vi "Begin.vi"(8 "error in":errorcluster) -> (0 "error out":errorcluster)   [LabVIEW 2017]
doc: "Called before other user functions, this VI is expected to open initial I/O refnums, load in file data, and do all program initialization. Notice that the <B>error out</B> terminal is simply used for data flow. Wiring it to other structures or subVIs ensures that this VI runs first."
uses:
  <vilib>/Rock Robotics/WPI/DriverStation/WPI_DriverStationRobotMode2.ctl
  <vilib>/Rock Robotics/SystemInterfaces/DIO/FPGA_DIOPWMChannel.ctl
  <vilib>/Rock Robotics/WPI/Joystick/WPI_JoystickDeviceEnum.ctl
  Robot Global Data.vi
  <vilib>/Rock Robotics/Network Tables/NT Write String Array.vi
  <vilib>/Rock Robotics/WPI/RobotDrive/WPI_RobotDriveOpen2MotorWithSPARK.vi
  <vilib>/Rock Robotics/WPI/RobotDrive/WPI_RobotDriveOpen4MotorWithSPARK.vi
  <vilib>/Rock Robotics/WPI/MotorControl/WPI_MotorControlOpen SPARK.vi
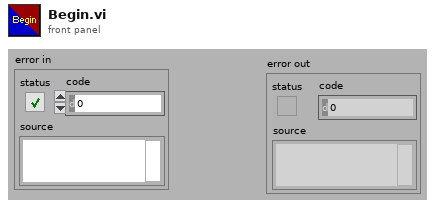
[diagram p1: front panel]
types:
  T1 = typedef "FPGA_DIOPWMChannel.ctl" = enum8{"PWM 0", "PWM 1", "PWM 2", "PWM 3", "PWM 4", "PWM 5", "PWM 6", "PWM 7", "PWM 8", "PWM 9", "PWM MXP 0", "PWM MXP 1", "PWM MXP 2", "PWM MXP 3", "PWM MXP 4", "PWM MXP 5", "PWM MXP 6", "PWM MXP 7", "PWM MXP 8", "PWM MXP 9", "Invalid"}
  T2 = typedef "WPI_JoystickDeviceEnum.ctl" = enum16{"USB 0", "USB 1", "USB 2", "USB 3", "USB 4", "USB 5"}
  T3 = typedef "WPI_DriverStationRobotMode2.ctl" = enum16{"Autonomous Disabled", "Autonomous Enabled", "Teleop Disabled", "Teleop Enabled", "Disconnected", "Finish", "Test Disabled", "Test Enabled", "Emergency Stopped"}
  T4 = typedef "WPI_MotorControlDeviceRef.ctl" = cluster{"DeviceStatus":errorcluster, "Type":T5, "PWM":cluster{"PWM Channel":T1, "DeadBand":T6}, "CAN":cluster{"Device Number":u8, "SetOutput VI Ref":variant, "GetOutput VI Ref":variant, "Enable VI Ref":variant, "Disable VI Ref":variant, "Data":variant}, "Invert":bool, "DIO PWM":cluster{"PWM \"Enable\" Channel":T1, "DIOChannel":T7, "PWM Rate":dbl}}
  T5 = typedef "WPI_MotorControlType.ctl" = enum16{"PWM", "CAN", "DIO PWM"}
  T6 = typedef "WPI_PWMDeadband.ctl" = cluster{"Name":string, "maxPositivePwm":i32, "minPositivePwm":i32, "centerPwm":i32, "maxNegativePwm":i32, "minNegativePwm":i32, "angularRange":u16}
  T7 = typedef "FPGA_DIOChannel.ctl" = enum8{"DIO 0", "DIO 1", "DIO 2", "DIO 3", "DIO 4", "DIO 5", "DIO 6", "DIO 7", "DIO 8", "DIO 9", "DIO MXP 0", "DIO MXP 1", "DIO MXP 2", "DIO MXP 3", "DIO MXP 4", "DIO MXP 5", "DIO MXP 6", "DIO MXP 7", "DIO MXP 8", "DIO MXP 9", "DIO MXP 10", "DIO MXP 11", "DIO MXP 12", "DIO MXP 13", "DIO MXP 14", "DIO MXP 15", "SPI Port CS1", "SPI Port CS2", "SPI Port CS3", "SPI Port MISO", "SPI Port MOSI", "Invalid"}
  T8 = typedef "WPI_RobotDriveDevRef.ctl" = cluster{"DevStatus":errorcluster, "Motors[]":T4[], "Square Inputs":bool, "Max Output":dbl}
  T9 = typedef "WPI_JoystickDevRef.ctl" = cluster{"Device":T2}
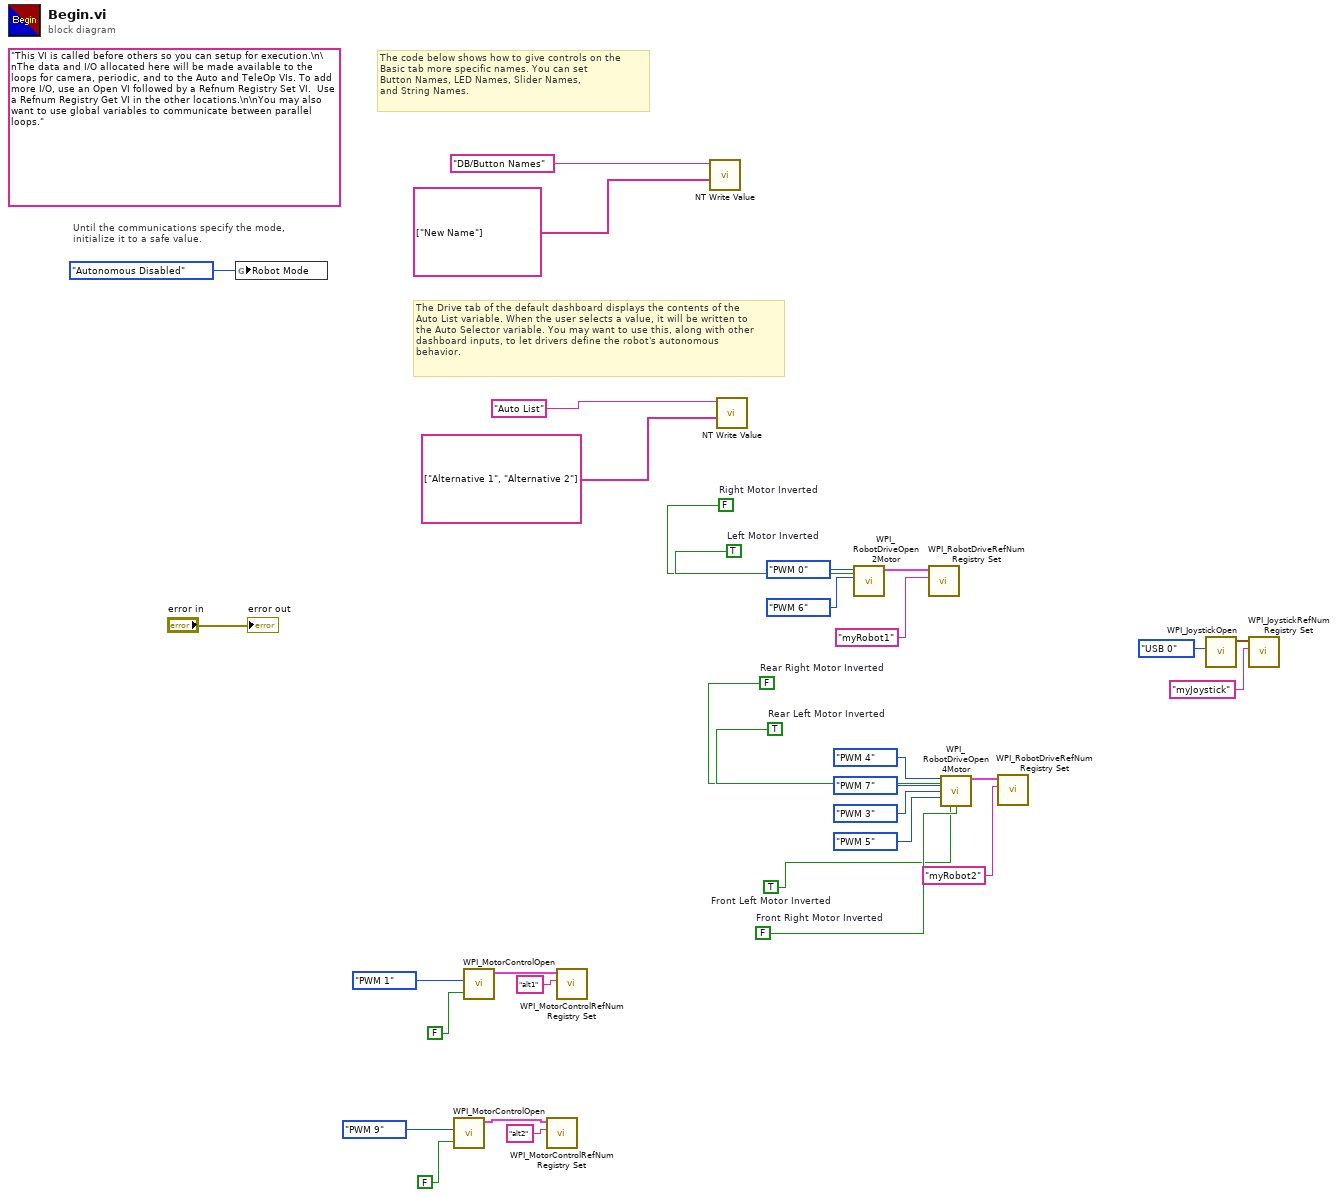
[diagram p0: block diagram]
diagram:
  w9 = TRUE  # Front Left Motor Inverted
  w10 = FALSE  # Front Right Motor Inverted
  w15 = FALSE  # Rear Right Motor Inverted
  w16 = TRUE  # Rear Left Motor Inverted
  w26 = FALSE  # Right Motor Inverted
  w27 = TRUE  # Left Motor Inverted
  (unwired) "This VI is called before others so you can setup for execution.\n\nThe data and I/O allocated here will be made available to the loops for camera, periodic, and to the Auto and TeleOp VIs. To add more I/O, use an Open VI followed by a Refnum Registry Set VI.  Use a Refnum Registry Get VI in the other locations.\n\nYou may also want to use global variables to communicate between parallel loops."
  # "The Drive tab of the default dashboard displays the contents of the\nAuto List variable. When the user selects a value, it will be written to\nthe Auto Selector variable. You may want to use this, along with other\ndashboard inputs, to let drivers define the robot's autonomous\nbehavior."
  # "The code below shows how to give controls on the\nBasic tab more specific names. You can set\nButton Names, LED Names, Slider Names,\nand String Names."
  # "Until the communications specify the mode,\ninitialize it to a safe value."
  n1 = global write "Robot Global Data.vi" "Robot Mode"(WPI_DriverStationRobotMode2."Autonomous Disabled" ("Robot Mode")) -> ()
  n2 = call-poly <vilib>:"WPI_MotorControlOpen.vi"("Invert"=FALSE, "PWM Channel"=FPGA_DIOPWMChannel."PWM 9") -> ("MotorControlDeviceRef"=w2:T4)  [unwired: 8 in, 1 out]
  n3 = call-poly <vilib>:"WPI_MotorControlOpen.vi"("Invert"=FALSE, "PWM Channel"=FPGA_DIOPWMChannel."PWM 1") -> ("MotorControlDeviceRef"=w6:T4)  [unwired: 8 in, 1 out]
  n4 = call <vilib>:"WPI_MotorControlRefNum Registry Set.vi"("refnum name"="alt2", "MotorControlDevRef"=w2) -> ()  [unwired: 8 in, 2 out]
  n5 = call <vilib>:"WPI_MotorControlRefNum Registry Set.vi"("refnum name"="alt1", "MotorControlDevRef"=w6) -> ()  [unwired: 8 in, 2 out]
  n6 = call-poly <vilib>:"NT Write Value.vi"("String Array"=string[] ["New Name"], "Name"="DB/Button Names") -> ()  [unwired: 9 in, 1 out]
  n7 = call-poly <vilib>:"NT Write Value.vi"("String Array"=string[] ["Alternative 1", "Alternative 2"], "Name"="Auto List") -> ()  [unwired: 9 in, 1 out]
  n8 = call-poly <vilib>:"WPI_RobotDriveOpen2Motor.vi"("Right Motor Inverted"=w26, "Left Motor Inverted"=w27, "Right Motor"=FPGA_DIOPWMChannel."PWM 6", "Left Motor"=FPGA_DIOPWMChannel."PWM 0") -> ("RobotDriveDevRef"=w24:T8)  [unwired: 6 in, 1 out]
  n9 = call <vilib>:"WPI_RobotDriveRefNum Registry Set.vi"("refnum name"="myRobot1", "RobotDriveDevRef"=w24) -> ()  [unwired: 8 in, 2 out]
  n10 = call-poly <vilib>:"WPI_RobotDriveOpen4Motor.vi"("Rear Left Motor"=FPGA_DIOPWMChannel."PWM 4", "Rear Left Motor Inverted"=w16, "Rear Right Motor Inverted"=w15, "Rear Right Motor"=FPGA_DIOPWMChannel."PWM 7", "Front Left Motor"=FPGA_DIOPWMChannel."PWM 3", "Front Right Motor"=FPGA_DIOPWMChannel."PWM 5", "Front Left Motor Inverted"=w9, "Front Right Motor Inverted"=w10) -> ("RobotDriveDevRef"=w18:T8)  [unwired: 6 in, 1 out]
  n11 = call <vilib>:"WPI_RobotDriveRefNum Registry Set.vi"("refnum name"="myRobot2", "RobotDriveDevRef"=w18) -> ()  [unwired: 8 in, 2 out]
  n12 = call <vilib>:"WPI_JoystickOpen.vi"("JoystickDevice"=WPI_JoystickDeviceEnum."USB 0") -> ("JoystickDevRef"=w20:T9)  [unwired: 10 in]
  n13 = call <vilib>:"WPI_JoystickRefNum Registry Set.vi"("refnum name"="myJoystick", "JoystickDevRef"=w20) -> ()  [unwired: 8 in, 2 out]
  "error out" <- "error in"
